vi "Measurement UI.vi"() -> ()   [LabVIEW 2021, in "adc_fullScaleError.lvlib"]
uses:
  adc_fullScaleError.lvlib
panel:
  in  "MeasGraphs":T1(tab)
  out "Negative Full Scale TransferFunction":cluster{"Waveform":dbl[], "DMM readings":dbl[]}(graph) caption="NegativeFullScaleGraph"
  out "Bipolar Zero TransferFunction":cluster{"Waveform":dbl[], "DMM readings":dbl[]}(graph) caption="BipolarZeroGraph"
  out "Positive Full Scale TransferFunction":cluster{"Waveform":dbl[], "DMM readings":dbl[]}(graph) caption="PositiveFullScaleGraph"
  out "ADC positive full scale readings":dbl[](array[numeric])
  out "ADC bipolar zero full scale readings":dbl[](array[numeric])
  out "ADC negative full scale readings":dbl[](array[numeric])
  out "DMM positive full scale readings":dbl[](array[numeric])
  out "DMM bipolar zero full scale readings":dbl[](array[numeric])
  out "DMM negative full scale readings":dbl[](array[numeric])
  out "Bipolar zero full scale error":dbl
  out "Negative full scale transition":dbl
  out "Positive full scale error":dbl
  out "Bipolar zero full scale transition":dbl
  out "Positive full scale transition":dbl
  out "Negative full scale error":dbl
  in  "DMM resource name":string
  out "Channel name":string
  in  "Analog source resource name":string
  in  "Digital capture resource name":string
  out "MeasTable":string[][](table)
  in  "DMM":string="DMM"
  in  "Digital capture":string="Digital capture"
  in  "Analog source":string="Analog source"
  in  "MeasSettingsOptions":i32(listbox)
  in  "MeasSettings":bool
  in  "Full scale range":dbl=10.0 caption="FULL SCALE RANGE" format="%#_6pV"
  in  "Transition step size":dbl=0.05 caption="TRANSITION STEP SIZE" format="%#_6gLSB"
  in  "Transition span":dbl=1.5 caption="TRANSITION SPAN" format="%#_6gLSB"
  in  "DMM resolution":dbl(ring)=5.5 caption="RESOLUTION IN DIGITS" items=["3 1/2"=3.5, "4 1/2"=4.5, "5 1/2"=5.5, "6 1/2"=6.5, "7 1/2"=7.5]
  in  "DMM range":dbl=10.0 caption="RANGE" format="%#_6pV"
  in  "DMMResourceName":refnum<k15> caption="RESOURCE NAME"
  in  "Digital capture samples":u32=10000 caption="NUMBER OF SAMPLES"
  in  "Input channel":i32=1 caption="INPUT CHANNEL" min=0 max=100 step=1
  in  "Digital capture sample rate":dbl=800000.0 caption="SAMPLE RATE" format="%#_6pS/s"
  in  "DSGResourceName":tag caption="RESOURCE NAME"
  in  "DPIResourceName":refnum<k15> caption="RESOURCE NAME"
  in  "ADC parameters":string="ADC parameters"
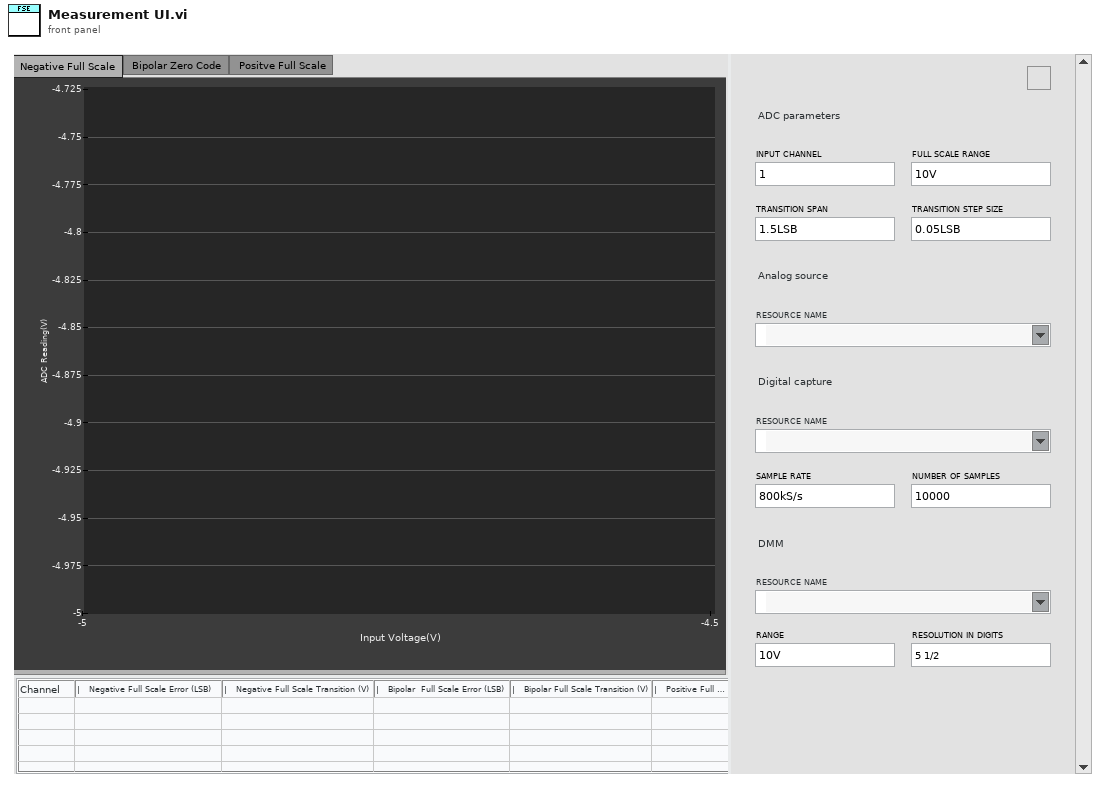
[diagram p1: front panel]
types:
  T1 = enum32{"Negative Full Scale ", "Bipolar Zero Code ", " Positve Full Scale", "Hidden Controls"}
  T2 = enum16{"open", "replace", "create", "open or create", "replace or create", "replace or create with confirmation"}
  T3 = cluster{"DMM negative full scale readings":dbl[], "ADC negative full scale readings":dbl[]}
  T4 = cluster{"DMM bipolar zero full scale readings":dbl[], "ADC bipolar zero full scale readings":dbl[]}
  T5 = cluster{"DMM positive full scale readings":dbl[], "ADC positive full scale readings":dbl[]}
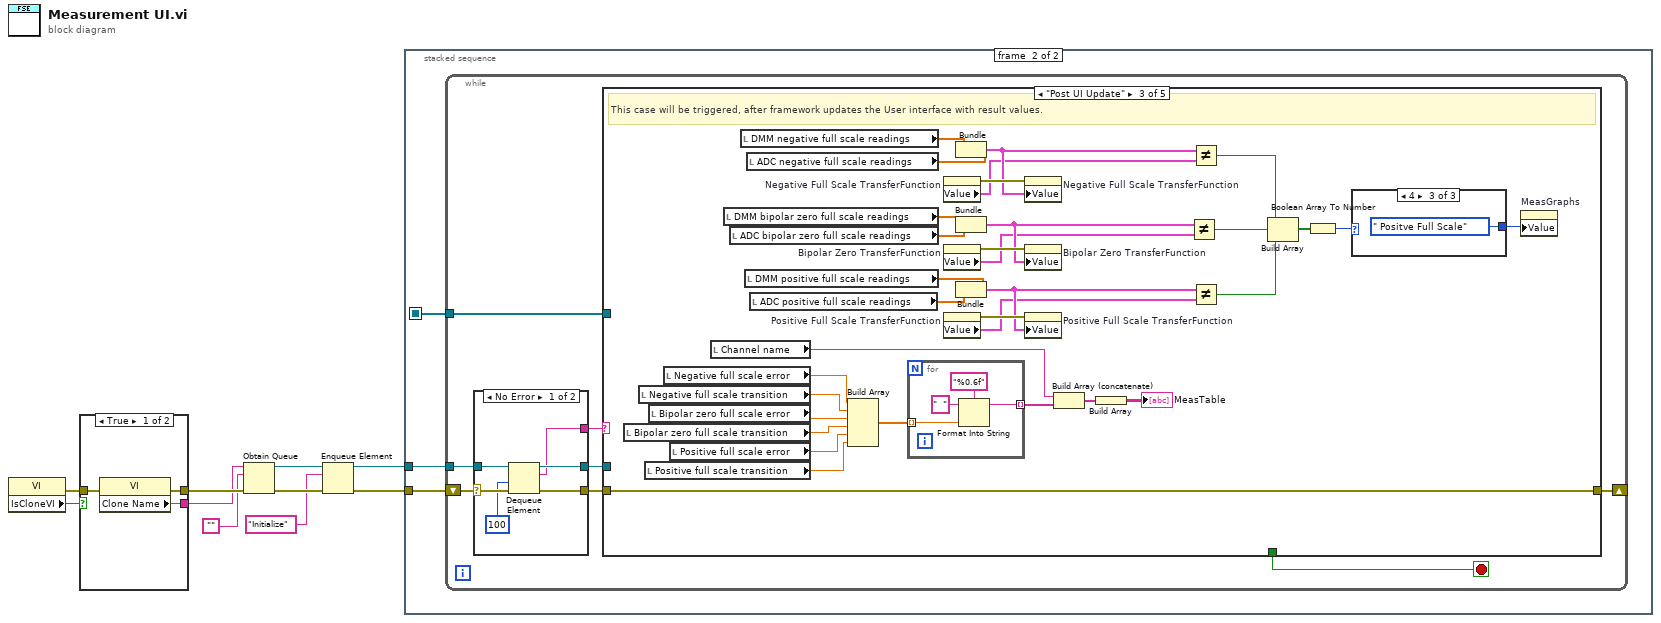
[diagram p0: block diagram]
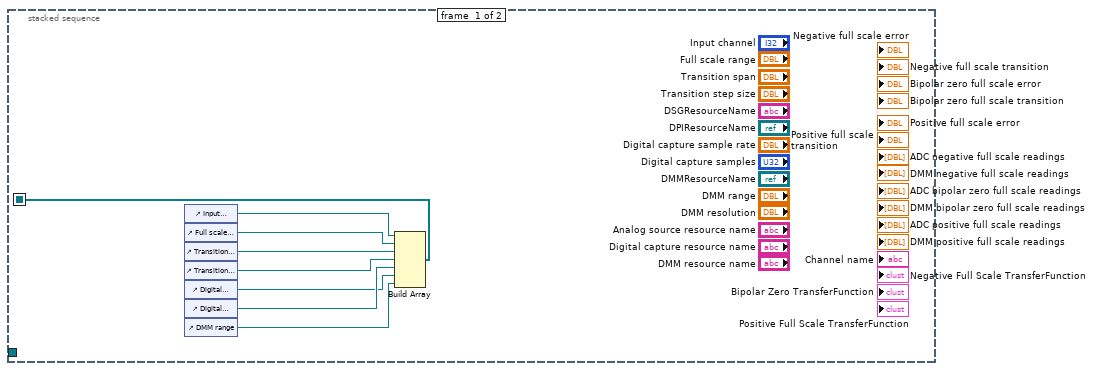
[diagram p2: hidden frame]
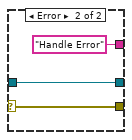
[diagram p3: hidden frame]
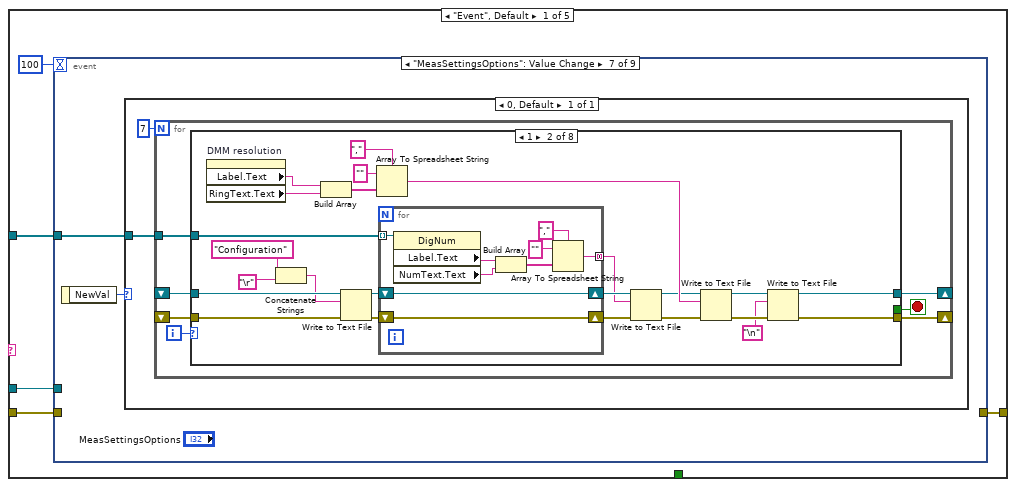
[diagram p4: hidden frame]
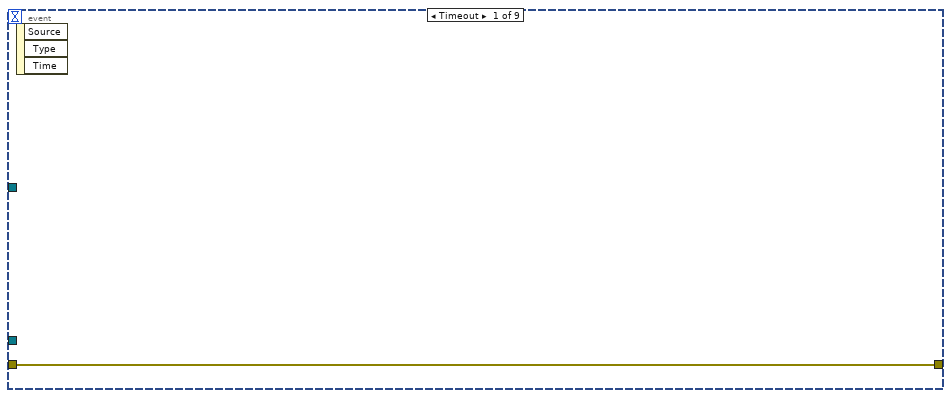
[diagram p5: hidden frame]
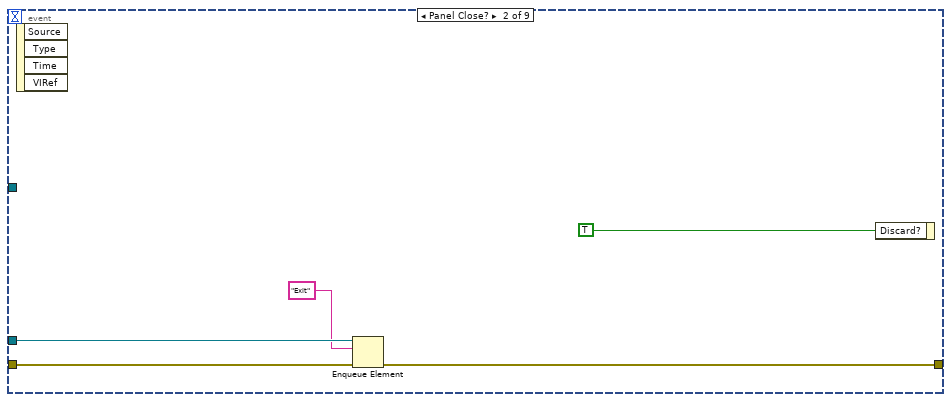
[diagram p6: hidden frame]
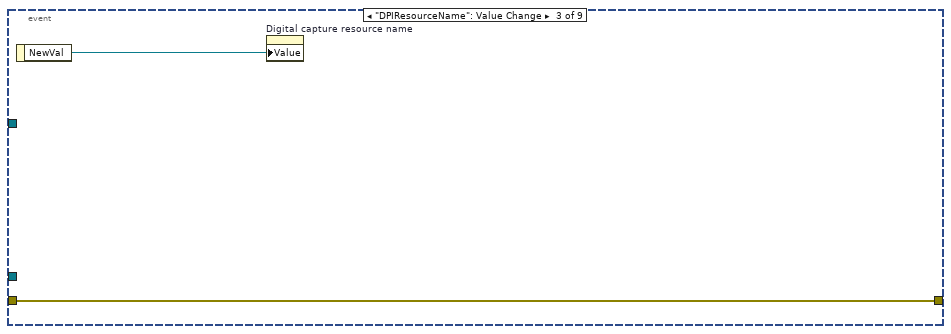
[diagram p7: hidden frame]
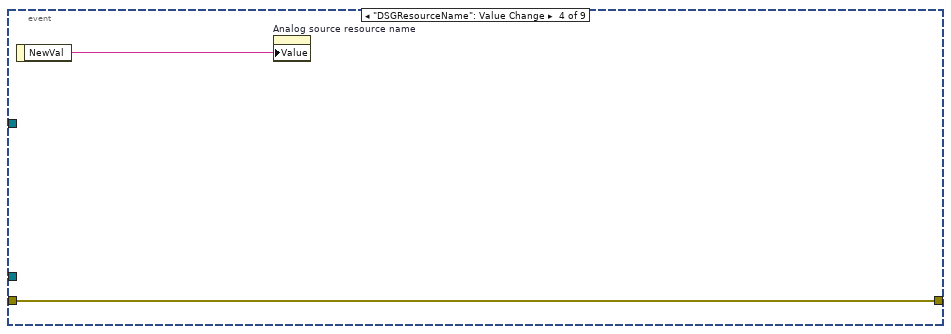
[diagram p8: hidden frame]
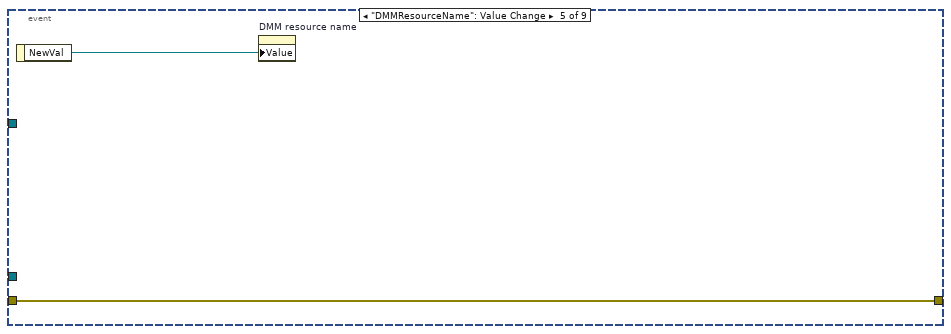
[diagram p9: hidden frame]
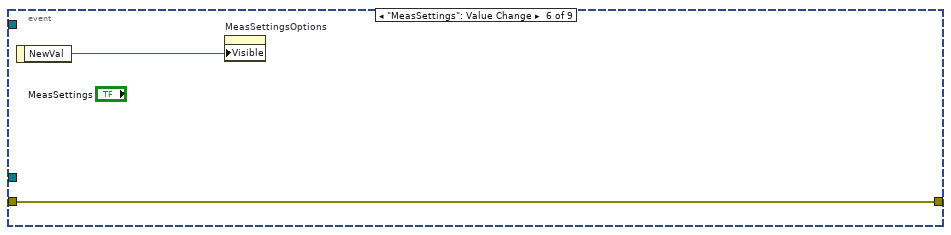
[diagram p10: hidden frame]
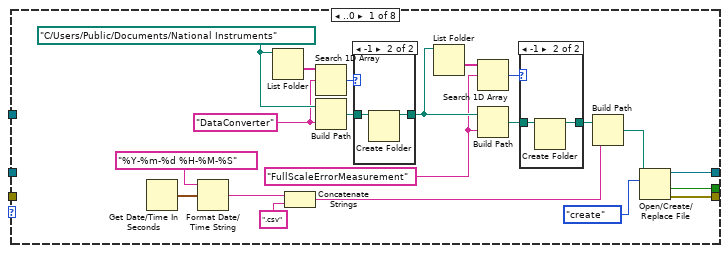
[diagram p11: hidden frame]
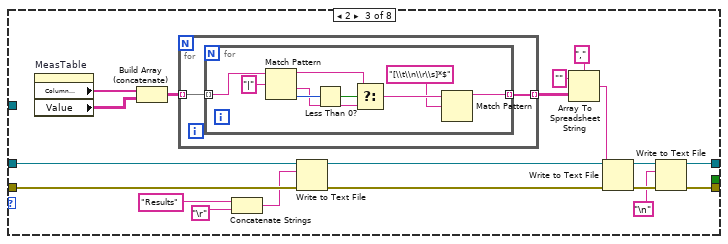
[diagram p14: hidden frame]
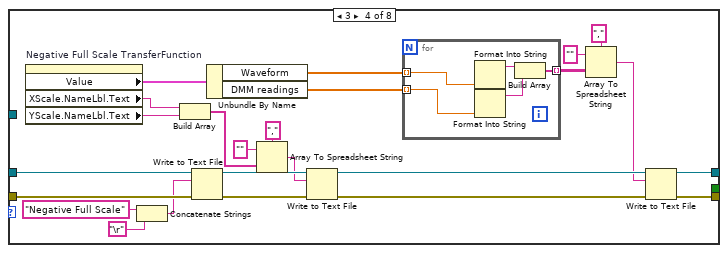
[diagram p15: hidden frame]
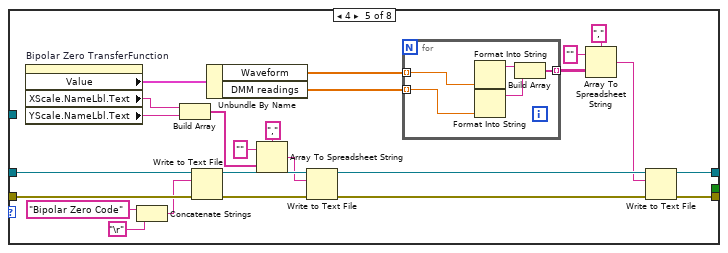
[diagram p16: hidden frame]
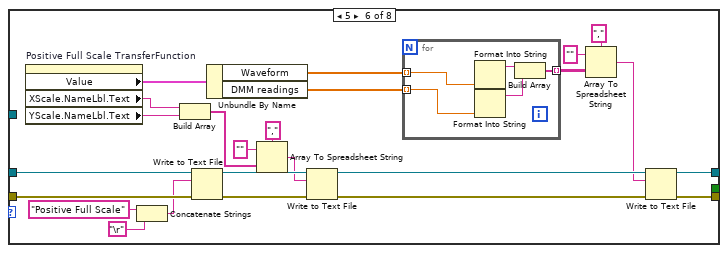
[diagram p17: hidden frame]
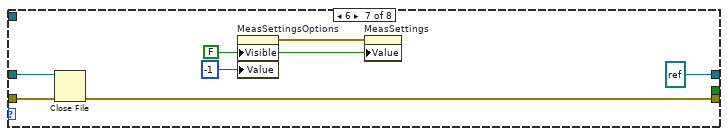
[diagram p18: hidden frame]
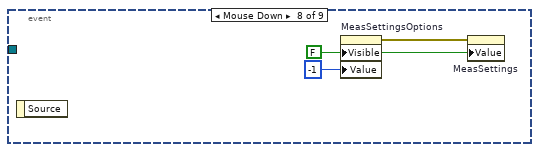
[diagram p20: hidden frame]
diagram:
  n1 = property class="VI"() -> (error out=w1:errorcluster, "IsCloneVI"=w2:bool)  [unwired: 2 in, 1 out]
  n2 = case shown="True" w2 {
    tunnel: [w13 w16] -> w10
    tunnel: [w12 w15] -> w9
    tunnel: w1 -> [w11 w14]
    frame True {
      n3 = property class="VI"(error in=w11) -> (error out=w13:errorcluster, "Clone Name"=w12:string)  [unwired: 1 in, 1 out]
    }
    frame False {
      n4 = property class="VI"(error in=w14) -> (error out=w16:errorcluster, "Name"=w15:string)  [unwired: 1 in, 1 out]
    }
  }
  n5 = Obtain Queue(name (unnamed)=w9, element data type="", error in (no error)=w10) -> (queue out=w6:refnum<queue>, error out=w8:errorcluster)  [unwired: 2 in, 1 out]
  n6 = Enqueue Element(queue=w6, element="Initialize", error in (no error)=w8) -> (queue out=w5:refnum<queue>, error out=w7:errorcluster)  [unwired: 1 in, 1 out]
  n7 = stacked-sequence {
    seq-local: [w17 _] -> [_ w25]
    tunnel: w7 -> [_ w27]
    tunnel: w5 -> [_ w26]
    frame #0 {
      n8 = control-ref of="Input channel"() -> (w24:refnum<vi>)
      n9 = control-ref of="Full scale range"() -> (w23:refnum<vi>)
      n10 = control-ref of="Transition span"() -> (w22:refnum<vi>)
      n11 = control-ref of="Transition step size"() -> (w21:refnum<vi>)
      n12 = control-ref of="Digital capture sample rate"() -> (w19:refnum<vi>)
      n13 = control-ref of="Digital capture samples"() -> (w20:refnum<vi>)
      n14 = control-ref of="DMM range"() -> (w18:refnum<vi>)
      n15 = Build Array(w24, w23, w22, w21, w20, w19, w18) -> (w17:refnum<vi>[])
    }
    frame #1 {
      n16 = while {
        shift-right: [w30] -> _
        shift-left: w27 -> [w35]
        tunnel: w26 -> [w33]
        tunnel: w25 -> [w28]
        stop <- w29 stop-if-true
        n17 = case shown="No Error" w35 {
          selector: w35 -> [w41 w44]
          tunnel: [w40 w44] -> w34
          tunnel: w33 -> [w39 w43]
          tunnel: [w38 w43] -> w32
          tunnel: [w37 "Handle Error"] -> w31
          frame No Error {
            n18 = Dequeue Element(queue=w39, timeout in ms (-1)=100, error in (no error)=w41) -> (queue out=w38:refnum<queue>, element=w37:string, error out=w40:errorcluster)  [unwired: 1 out]
          }
          frame Error {
          }
        }
        n19 = case shown="\"Post UI Update\"" w31 {
          tunnel: w34 -> [w48 w285 w320 w334 w335]
          tunnel: w32 -> [w46 _ _ w332 _]
          tunnel: [w49 w285 w320 w329 w335] -> w30
          tunnel: [_ FALSE _ TRUE _] -> w29
          tunnel: w28 -> [w45 _ _ _ _]
          frame "Event", Default {
            n20 = event shown="[6] \"MeasSettingsOptions\": Value Change" {
              selector: _ -> [_ _ _ _ _ _ _ _ _]
              dyn-events: _ -> [_ _ _ _ _ _ _ _ _]
              timeout: 100 -> [_ _ _ _ _ _ _ _ _]
              tunnel: [w50 w53 w56 w58 w61 w63 _ _ w264] -> w49
              tunnel: w48 -> [w50 w54 w56 w58 w61 w63 _ _ w264]
              tunnel: w46 -> [_ w52 _ _ _ _ _ _ _]
              tunnel: w45 -> [_ _ _ _ _ _ w64 _ _]
              event Timeout {
                n21 = event-data() -> ()  [unwired: 1 in, 3 out]
              }
              event Panel Close? {
                n22 = event-data() -> ()  [unwired: 1 in, 4 out]
                n23 = Enqueue Element(queue=w52, element="Exit", error in (no error)=w54) -> (error out=w53:errorcluster)  [unwired: 1 in, 2 out]
                n24 = event-data("Discard?"=TRUE) -> ()  [unwired: 1 in, 1 out]
              }
              event "DPIResourceName": Value Change {
                n25 = event-data() -> ("NewVal"=w57:refnum<k15>)  [unwired: 1 in]
                n26 = property on="Digital capture resource name" class="Str"("Value"=w57) -> ()  [unwired: 2 in, 2 out]
              }
              event "DSGResourceName": Value Change {
                n27 = event-data() -> ("NewVal"=w59:tag)  [unwired: 1 in]
                n28 = property on="Analog source resource name" class="Str"("Value"=w59) -> ()  [unwired: 2 in, 2 out]
              }
              event "DMMResourceName": Value Change {
                n29 = event-data() -> ("NewVal"=w60:refnum<k15>)  [unwired: 1 in]
                n30 = property on="DMM resource name" class="Str"("Value"=w60) -> ()  [unwired: 2 in, 2 out]
              }
              event "MeasSettings": Value Change {
                n31 = event-data() -> ("NewVal"=w62:bool)  [unwired: 1 in]
                n32 = property on="MeasSettingsOptions" class="LstBox (strict)"("Visible"=w62) -> ()  [unwired: 2 in, 2 out]
              }
              event "MeasSettingsOptions": Value Change {
                n33 = event-data() -> ("NewVal"=w65:i32)  [unwired: 1 in]
                n34 = case shown="0, Default" w65 {
                  tunnel: w64 -> [w66]
                  frame 0, Default {
                    n35 = for {
                      N: 7 -> [_]
                      shift-right: [w72] -> _
                      shift-left: _ -> [w71]
                      shift-right: [w70] -> _
                      shift-left: _ -> [w69]
                      tunnel: w66 -> [w68]
                      i -> [w74]
                      stop <- w73 stop-if-true
                      n36 = case shown="1" w74 {
                        tunnel: [w88 _ _ _ _ _ _ _] -> w73
                        tunnel: [w94 w107 w142 w177 w206 w235 refnum<file> refnum ("refnum out") w260] -> w72
                        tunnel: w71 -> [_ w123 w153 w188 w217 w246 w255 w260]
                        tunnel: [w87 w105 w141 w176 w205 w234 w253 w259] -> w70
                        tunnel: w69 -> [_ w121 w152 w187 w216 w245 w254 w259]
                        tunnel: w68 -> [_ w125 _ _ _ _ _ _]
                        frame ..0 {
                          w83 = "FullScaleErrorMeasurement" ("prompt")
                          w90 = "DataConverter" ("prompt")
                          w93 = path "C:/Users/Public/Documents/National Instruments" ("base path")
                          n37 = Get Date/Time In Seconds() -> (seconds since 1Jan1904=w80:timestamp)
                          n38 = Format Date/Time String(time format string (%c)="%Y-%m-%d %H-%M-%S", seconds (now)=w80) -> (date/time string=w79:string)  [unwired: 1 in]
                          n39 = List Folder(path=w93) -> (folder names=w91:string[])  [unwired: 3 in, 3 out]
                          n40 = Concatenate Strings(w79, ".csv" ("string")) -> (w76:string)
                          n41 = Search 1D Array(1D array=w91, element=w90) -> (index of element=w89:i32)  [unwired: 1 in]
                          n42 = Build Path(base path=w93, name or relative path=w90) -> (appended path=w92:path)
                          n43 = case shown="-1" w89 {
                            tunnel: w92 -> [w99 w101]
                            tunnel: [w99 w100] -> w84
                            frame Default {
                            }
                            frame -1 {
                              n44 = Create Folder(path (use dialog)=w101) -> (created path=w100:path)  [unwired: 2 in, 2 out]
                            }
                          }
                          n45 = List Folder(path=w84) -> (folder names=w86:string[])  [unwired: 3 in, 3 out]
                          n46 = Search 1D Array(1D array=w86, element=w83) -> (index of element=w85:i32)  [unwired: 1 in]
                          n47 = Build Path(base path=w84, name or relative path=w83) -> (appended path=w82:path)
                          n48 = case shown="-1" w85 {
                            tunnel: w82 -> [w96 w98]
                            tunnel: [w96 w97] -> w77
                            frame Default {
                            }
                            frame -1 {
                              n49 = Create Folder(path (use dialog)=w98) -> (created path=w97:path)  [unwired: 2 in, 2 out]
                            }
                          }
                          n50 = Build Path(base path=w77, name or relative path=w76) -> (appended path=w75:path)
                          n51 = Open/Create/Replace File(file path (use dialog)=w75, operation (0:open)=T2."create") -> (refnum out=w94:refnum<file>, cancelled=w88:bool, error out=w87:errorcluster)  [unwired: 4 in]
                        }
                        frame 1 {
                          n52 = property on="DMM resolution" class="Ring (strict)"() -> ("Label.Text"=w103:string, "RingText.Text"=w102:string)  [unwired: 2 in, 2 out]
                          n53 = Concatenate Strings("Configuration" ("format string"), "\r") -> (w118:string)
                          n54 = Build Array(w103, w102) -> (w115:string[])
                          n55 = Write to Text File(file (use dialog)=w123, text=w118, error in=w121) -> (refnum out=w124:refnum<file>, error out=w122:errorcluster)  [unwired: 1 in, 1 out]
                          n56 = Array To Spreadsheet String(delimiter (Tab)=",", array=w115, 3:"" ("format string")) -> (spreadsheet string=w114:string)
                          n57 = for {
                            tunnel: w125 -> [w134] mode=indexing
                            shift-right: [w131] -> w113
                            shift-left: w124 -> [w131]
                            shift-right: [w130] -> w111
                            shift-left: w122 -> [w130]
                            tunnel: [w126] -> w109 mode=concatenating
                            n58 = property class="DigNum"(reference=w134) -> ("Label.Text"=w133:string, "NumText.Text"=w132:string)  [unwired: 1 in, 2 out]
                            n59 = Build Array(w133, w132) -> (w127:string[])
                            n60 = Array To Spreadsheet String(delimiter (Tab)=",", array=w127, 3:"" ("format string")) -> (spreadsheet string=w126:string)
                          }
                          n61 = Write to Text File(file (use dialog)=w113, text=w109, error in=w111) -> (refnum out=w112:refnum<file>, error out=w110:errorcluster)  [unwired: 1 in, 1 out]
                          n62 = Write to Text File(file (use dialog)=w112, text=w114, error in=w110) -> (refnum out=w108:refnum<file>, error out=w106:errorcluster)  [unwired: 1 in, 1 out]
                          n63 = Write to Text File(file (use dialog)=w108, text="\n", error in=w106) -> (refnum out=w107:refnum<file>, error out=w105:errorcluster)  [unwired: 1 in, 1 out]
                        }
                        frame 2 {
                          n64 = property on="MeasTable" class="Tbl (strict)"() -> ("Column Headers[]"=w136:string[], "Value"=w135:string[][])  [unwired: 2 in, 2 out]
                          n65 = Build Array (concatenate)(w136, w135) -> (w150:string[][])
                          n66 = for {
                            tunnel: w150 -> [w155] mode=indexing
                            tunnel: [w154] -> w149 mode=indexing
                            n67 = for {
                              tunnel: w155 -> [w157] mode=indexing
                              tunnel: [w156] -> w154 mode=indexing
                              n68 = Match Pattern(string=w157, regular expression="|") -> (before substring=w161:string, after substring=w160:string, offset past match=w163:i32)  [unwired: 1 in, 1 out]
                              n69 = Less Than 0?(x=w163) -> (x < 0?=w162:bool)
                              n70 = Select(t=w161, s=w162, f=w160) -> (s? t:f=w159:string)
                              n71 = Match Pattern(string=w159, regular expression="[\\t\\n\\r\\s]*$") -> (before substring=w156:string)  [unwired: 1 in, 3 out]
                            }
                          }
                          n72 = Concatenate Strings("Results" ("element"), "\r") -> (w137:string)
                          n73 = Write to Text File(file (use dialog)=w153, text=w137, error in=w152) -> (refnum out=w151:refnum<file>, error out=w145:errorcluster)  [unwired: 1 in, 1 out]
                          n74 = Array To Spreadsheet String(delimiter (Tab)=",", array=w149, 3:"" ("format string")) -> (spreadsheet string=w146:string)
                          n75 = Write to Text File(file (use dialog)=w151, text=w146, error in=w145) -> (refnum out=w144:refnum<file>, error out=w143:errorcluster)  [unwired: 1 in, 1 out]
                          n76 = Write to Text File(file (use dialog)=w144, text="\n", error in=w143) -> (refnum out=w142:refnum<file>, error out=w141:errorcluster)  [unwired: 1 in, 1 out]
                        }
                        frame 3 {
                          n77 = property on="Negative Full Scale TransferFunction" class="XYGraph (strict)"() -> ("Value"=w168:cluster{"Waveform":dbl[], "DMM readings":dbl[]}, "XScale.NameLbl.Text"=w167:string, "YScale.NameLbl.Text"=w166:string)  [unwired: 2 in, 2 out]
                          n78 = Concatenate Strings("Negative Full Scale" ("string"), "\r") -> (w185:string)
                          n79 = Build Array(w167, w166) -> (w165:string[])
                          n80 = Write to Text File(file (use dialog)=w188, text=w185, error in=w187) -> (refnum out=w182:refnum<file>, error out=w181:errorcluster)  [unwired: 1 in, 1 out]
                          n81 = Unbundle By Name(w168) -> ("Waveform"=w171:dbl[], "DMM readings"=w172:dbl[])
                          n82 = Array To Spreadsheet String(delimiter (Tab)=",", array=w165, 3:"" ("format string")) -> (spreadsheet string=w180:string)
                          n83 = Write to Text File(file (use dialog)=w182, text=w180, error in=w181) -> (refnum out=w179:refnum<file>, error out=w178:errorcluster)  [unwired: 1 in, 1 out]
                          n84 = for {
                            tunnel: w171 -> [w190] mode=indexing
                            tunnel: w172 -> [w189] mode=indexing
                            tunnel: [w191] -> w173 mode=indexing
                            n85 = Format Into String(w190) -> (resulting string=w192:string)  [unwired: 3 in, 1 out]
                            n86 = Format Into String(w189) -> (resulting string=w193:string)  [unwired: 3 in, 1 out]
                            n87 = Build Array(w192, w193) -> (w191:string[])
                          }
                          n88 = Array To Spreadsheet String(delimiter (Tab)=",", array=w173, 3:"" ("format string")) -> (spreadsheet string=w170:string)
                          n89 = Write to Text File(file (use dialog)=w179, text=w170, error in=w178) -> (refnum out=w177:refnum<file>, error out=w176:errorcluster)  [unwired: 1 in, 1 out]
                        }
                        frame 4 {
                          n90 = property on="Bipolar Zero TransferFunction" class="XYGraph (strict)"() -> ("Value"=w197:cluster{"Waveform":dbl[], "DMM readings":dbl[]}, "XScale.NameLbl.Text"=w196:string, "YScale.NameLbl.Text"=w195:string)  [unwired: 2 in, 2 out]
                          n91 = Concatenate Strings("Bipolar Zero Code" ("string"), "\r") -> (w214:string)
                          n92 = Build Array(w196, w195) -> (w194:string[])
                          n93 = Write to Text File(file (use dialog)=w217, text=w214, error in=w216) -> (refnum out=w211:refnum<file>, error out=w210:errorcluster)  [unwired: 1 in, 1 out]
                          n94 = Unbundle By Name(w197) -> ("Waveform"=w200:dbl[], "DMM readings"=w201:dbl[])
                          n95 = Array To Spreadsheet String(delimiter (Tab)=",", array=w194, 3:"" ("format string")) -> (spreadsheet string=w209:string)
                          n96 = Write to Text File(file (use dialog)=w211, text=w209, error in=w210) -> (refnum out=w208:refnum<file>, error out=w207:errorcluster)  [unwired: 1 in, 1 out]
                          n97 = for {
                            tunnel: w200 -> [w219] mode=indexing
                            tunnel: w201 -> [w218] mode=indexing
                            tunnel: [w220] -> w202 mode=indexing
                            n98 = Format Into String(w219) -> (resulting string=w221:string)  [unwired: 3 in, 1 out]
                            n99 = Format Into String(w218) -> (resulting string=w222:string)  [unwired: 3 in, 1 out]
                            n100 = Build Array(w221, w222) -> (w220:string[])
                          }
                          n101 = Array To Spreadsheet String(delimiter (Tab)=",", array=w202, 3:"" ("format string")) -> (spreadsheet string=w199:string)
                          n102 = Write to Text File(file (use dialog)=w208, text=w199, error in=w207) -> (refnum out=w206:refnum<file>, error out=w205:errorcluster)  [unwired: 1 in, 1 out]
                        }
                        frame 5 {
                          n103 = property on="Positive Full Scale TransferFunction" class="XYGraph (strict)"() -> ("Value"=w226:cluster{"Waveform":dbl[], "DMM readings":dbl[]}, "XScale.NameLbl.Text"=w225:string, "YScale.NameLbl.Text"=w224:string)  [unwired: 2 in, 2 out]
                          n104 = Concatenate Strings("Positive Full Scale" ("string"), "\r") -> (w243:string)
                          n105 = Build Array(w225, w224) -> (w223:string[])
                          n106 = Write to Text File(file (use dialog)=w246, text=w243, error in=w245) -> (refnum out=w240:refnum<file>, error out=w239:errorcluster)  [unwired: 1 in, 1 out]
                          n107 = Unbundle By Name(w226) -> ("Waveform"=w229:dbl[], "DMM readings"=w230:dbl[])
                          n108 = Array To Spreadsheet String(delimiter (Tab)=",", array=w223, 3:"" ("format string")) -> (spreadsheet string=w238:string)
                          n109 = Write to Text File(file (use dialog)=w240, text=w238, error in=w239) -> (refnum out=w237:refnum<file>, error out=w236:errorcluster)  [unwired: 1 in, 1 out]
                          n110 = for {
                            tunnel: w229 -> [w248] mode=indexing
                            tunnel: w230 -> [w247] mode=indexing
                            tunnel: [w249] -> w231 mode=indexing
                            n111 = Format Into String(w248) -> (resulting string=w250:string)  [unwired: 3 in, 1 out]
                            n112 = Format Into String(w247) -> (resulting string=w251:string)  [unwired: 3 in, 1 out]
                            n113 = Build Array(w250, w251) -> (w249:string[])
                          }
                          n114 = Array To Spreadsheet String(delimiter (Tab)=",", array=w231, 3:"" ("format string")) -> (spreadsheet string=w228:string)
                          n115 = Write to Text File(file (use dialog)=w237, text=w228, error in=w236) -> (refnum out=w235:refnum<file>, error out=w234:errorcluster)  [unwired: 1 in, 1 out]
                        }
                        frame 6 {
                          w257 = FALSE ("Visible")
                          n116 = Close File(refnum=w255, error in=w254) -> (error out=w253:errorcluster)  [unwired: 1 out]
                          n117 = property on="MeasSettingsOptions" class="LstBox (strict)"("Visible"=w257, "Value"=-1 ("MeasSettingsOptions")) -> (error out=w258:errorcluster)  [unwired: 2 in, 1 out]
                          n118 = property on="MeasSettings" class="Bool (strict)"(error in=w258, "Value"=w257) -> ()  [unwired: 1 in, 2 out]
                        }
                        frame Default {
                        }
                      }
                    }
                  }
                }
              }
              event Mouse Down {
                w262 = FALSE ("Visible")
                n119 = event-data() -> ()  [unwired: 1 in, 1 out]
                n120 = property on="MeasSettingsOptions" class="LstBox (strict)"("Visible"=w262, "Value"=-1 ("MeasSettingsOptions")) -> (error out=w263:errorcluster)  [unwired: 2 in, 1 out]
                n121 = property on="MeasSettings" class="Bool (strict)"(error in=w263, "Value"=w262) -> ()  [unwired: 1 in, 2 out]
              }
              event "Negative Full Scale TransferFunction", "Bipolar Zero TransferFunction", "Positive Full Scale TransferFunction": Shortcut Menu Selection (User) {
                n122 = event-data() -> ("ItemTag"=w268:string)  [unwired: 1 in]
                n123 = case shown="\" Positve Full Scale\"" "MeasGraphs" {
                  tunnel: [w269 w270 w271] -> w266
                  frame "Negative Full Scale ", Default {
                    n124 = control-ref of="Negative Full Scale TransferFunction"() -> (w269:refnum<vi>)
                  }
                  frame "Bipolar Zero Code " {
                    n125 = control-ref of="Bipolar Zero TransferFunction"() -> (w270:refnum<vi>)
                  }
                  frame " Positve Full Scale" {
                    n126 = control-ref of="Positive Full Scale TransferFunction"() -> (w271:refnum<vi>)
                  }
                }
                n127 = case shown="\"ZOOM_TO_RECTANGLE\", Default" w268 {
                  tunnel: [2 ("Palette:Active Tool") 3 ("Palette:Active Tool") 4 ("Palette:Active Tool") 5 ("Palette:Active Tool") 1 ("Palette:Active Tool")] -> w265
                  frame "ZOOM_TO_RECTANGLE", Default {
                  }
                  frame "X_ZOOM" {
                  }
                  frame "Y_ZOOM" {
                  }
                  frame "ZOOM_TO_FIT" {
                  }
                  frame "PANNING_TOOL" {
                  }
                }
                n128 = property class="XYGraph (strict)"(reference=w266, "ActPaletteTool"=w265) -> ()  [unwired: 1 in, 2 out]
              }
            }
          }
          frame "Initialize" {
            w278 = 2 ("Palette:Active Tool")
            w279 = string[] ["Export data"] ("Item Names")
            w283 = "<Select Device>"
            n129 = property on="Negative Full Scale TransferFunction" class="XYGraph (strict)"("ActPaletteTool"=w278) -> ()  [unwired: 2 in, 2 out]
            n130 = property on="MeasSettingsOptions" class="LstBox (strict)"("Item Names"=w279, "Value"=-1 ("MeasSettingsOptions"), "Visible"=FALSE, "Disabled Items"=i32[] []) -> ()  [unwired: 2 in, 2 out]
            n131 = property on="Bipolar Zero TransferFunction" class="XYGraph (strict)"("ActPaletteTool"=w278) -> ()  [unwired: 2 in, 2 out]
            n132 = property on="DPIResourceName" class="IVIName"("Value"=w283) -> ()  [unwired: 2 in, 2 out]
            n133 = property on="DSGResourceName" class="DAQmxName"("Value"=w283) -> ()  [unwired: 2 in, 2 out]
            n134 = property on="DMMResourceName" class="IVIName"("Value"=w283) -> ()  [unwired: 2 in, 2 out]
            n135 = property on="Positive Full Scale TransferFunction" class="XYGraph (strict)"("ActPaletteTool"=w278) -> ()  [unwired: 2 in, 2 out]
            n136 = for {
              tunnel: w279 -> [_] mode=indexing
              i -> [w287]
              n137 = property on="MeasSettingsOptions" class="LstBox (strict)"("Active Row"=w287, "Cell Height"=30 ("Active Row:Cell Height")) -> ()  [unwired: 2 in, 2 out]
            }
            n138 = property on="MeasGraphs" class="TabCtl (strict)"("Value"=T1."Negative Full Scale " ("MeasGraphs")) -> ()  [unwired: 2 in, 2 out]
          }
          frame "Post UI Update" {
            # "This case will be triggered, after framework updates the User interface with result values."
            n139 = local read "Bipolar zero full scale transition"() -> (w314:dbl)
            n140 = local read "Negative full scale transition"() -> (w316:dbl)
            n141 = local read "Positive full scale transition"() -> (w312:dbl)
            n142 = local read "Bipolar zero full scale error"() -> (w315:dbl)
            n143 = local read "Negative full scale error"() -> (w318:dbl)
            n144 = local read "Positive full scale error"() -> (w313:dbl)
            n145 = local read "Channel name"() -> (w317:string)
            n146 = local read "DMM bipolar zero full scale readings"() -> (w306:dbl[])
            n147 = local read "ADC bipolar zero full scale readings"() -> (w307:dbl[])
            n148 = local read "DMM negative full scale readings"() -> (w309:dbl[])
            n149 = local read "DMM positive full scale readings"() -> (w304:dbl[])
            n150 = local read "ADC negative full scale readings"() -> (w308:dbl[])
            n151 = local read "ADC positive full scale readings"() -> (w305:dbl[])
            n152 = Build Array(w318, w316, w315, w314, w313, w312) -> (w311:dbl[])
            n153 = for {
              tunnel: w311 -> [w327] mode=indexing
              tunnel: [w324] -> w310 mode=indexing
              n154 = Format Into String(format string="%0.6f", initial string="  ", w327) -> (resulting string=w324:string)  [unwired: 1 in, 1 out]
            }
            n155 = property on="Negative Full Scale TransferFunction" class="XYGraph (strict)"() -> (error out=w297:errorcluster, "Value"=w295:cluster{"Waveform":dbl[], "DMM readings":dbl[]})  [unwired: 2 in, 1 out]
            n156 = property on="Bipolar Zero TransferFunction" class="XYGraph (strict)"() -> (error out=w294:errorcluster, "Value"=w292:cluster{"Waveform":dbl[], "DMM readings":dbl[]})  [unwired: 2 in, 1 out]
            n157 = property on="Positive Full Scale TransferFunction" class="XYGraph (strict)"() -> (error out=w290:errorcluster, "Value"=w288:cluster{"Waveform":dbl[], "DMM readings":dbl[]})  [unwired: 2 in, 1 out]
            n158 = Bundle("DMM negative full scale readings"=w309, "ADC negative full scale readings"=w308) -> (w296:T3)  [unwired: 1 in]
            n159 = Bundle("DMM bipolar zero full scale readings"=w306, "ADC bipolar zero full scale readings"=w307) -> (w293:T4)  [unwired: 1 in]
            n160 = Bundle("DMM positive full scale readings"=w304, "ADC positive full scale readings"=w305) -> (w289:T5)  [unwired: 1 in]
            n161 = property on="Negative Full Scale TransferFunction" class="XYGraph (strict)"(error in=w297, "Value"=w296) -> ()  [unwired: 1 in, 2 out]
            n162 = property on="Bipolar Zero TransferFunction" class="XYGraph (strict)"(error in=w294, "Value"=w293) -> ()  [unwired: 1 in, 2 out]
            n163 = property on="Positive Full Scale TransferFunction" class="XYGraph (strict)"(error in=w290, "Value"=w289) -> ()  [unwired: 1 in, 2 out]
            n164 = Build Array (concatenate)(w317, w310) -> (w319:string[])
            n165 = Build Array(w319) -> (→"MeasTable":string[][])
            n166 = Not Equal?(x=w293, y=w292) -> (x != y?=w291:bool)
            n167 = Not Equal?(x=w296, y=w295) -> (x != y?=w302:bool)
            n168 = Not Equal?(x=w289, y=w288) -> (x != y?=w301:bool)
            n169 = Build Array(w302, w291, w301) -> (w300:bool[])
            n170 = Boolean Array To Number(Boolean array=w300) -> (number=w299:u32)
            n171 = case shown="4" w299 {
              tunnel: [T1."Negative Full Scale " ("MeasGraphs") T1."Bipolar Zero Code " ("MeasGraphs") T1." Positve Full Scale" ("MeasGraphs")] -> w298
              frame 1, Default {
              }
              frame 2 {
              }
              frame 4 {
              }
            }
            n172 = property on="MeasGraphs" class="TabCtl (strict)"("Value"=w298) -> ()  [unwired: 2 in, 2 out]
          }
          frame "Exit" {
            # "This case is triggered to close the User Interface from framework"
            n173 = Flush Queue(queue=w332, error in (no error)=w334) -> (queue out=w331:refnum<queue>, error out=w330:errorcluster)  [unwired: 1 out]
            n174 = Release Queue(queue=w331, force destroy? (F)=TRUE, error in (no error)=w330) -> (error out=w329:errorcluster)  [unwired: 2 out]
          }
          frame "Handle Error" {
          }
        }
      }
    }
  }
